vi "Parse U64 Ind Regs.vi"(9 "ECUEvents In":T2, 10 "APU Registers In":T4, 11 "U64":T3[](array[typedef])) -> (1 "ECUEvents Out":T2, 2 "APU Registers Out":T4)   [LabVIEW 2011, in "Engine Sim System Explorer.lvlib"]
uses:
  Engine Sim System Explorer.lvlib
  TypeDefs/APUComp.ctl
  TypeDefs/ECUEventRegs.ctl
  <userlib>/_FPGA Interface Advanced Tools/FPGA Bitfile Utility/TypeDefs/Scalar Register.ctl
  <userlib>/_FPGA Interface Advanced Tools/FPGA Bitfile Utility/FPGA Bitfile Utility.lvlib
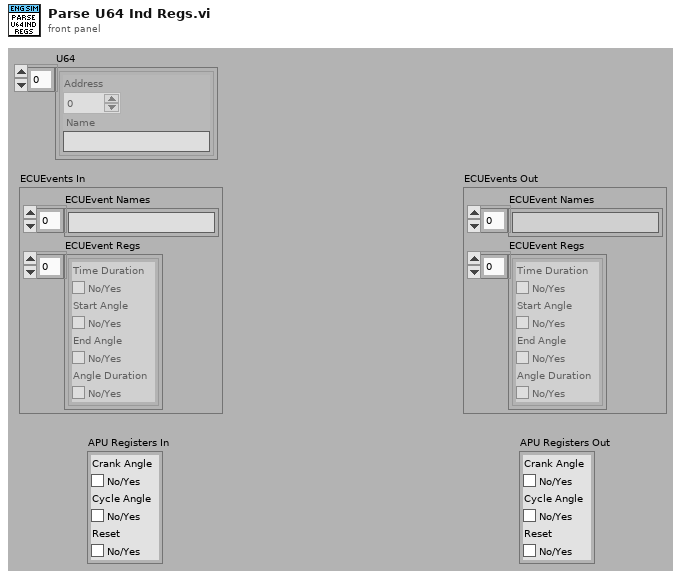
[diagram p1: front panel]
types:
  T1 = typedef "Engine Sim System Explorer.lvlib/ECUEventRegs.ctl" = cluster{"Time Duration":bool, "Start Angle":bool, "End Angle":bool, "Angle Duration":bool}
  T2 = cluster{"ECUEvent Names":string[], "ECUEvent Regs":T1[]}
  T3 = typedef "FPGA Bitfile Utility.lvlib/Scalar Register.ctl" = cluster{"Address":u32, "Name":string}
  T4 = typedef "Engine Sim System Explorer.lvlib/APUComp.ctl" = cluster{"Crank Angle":bool, "Cycle Angle":bool, "Reset":bool}
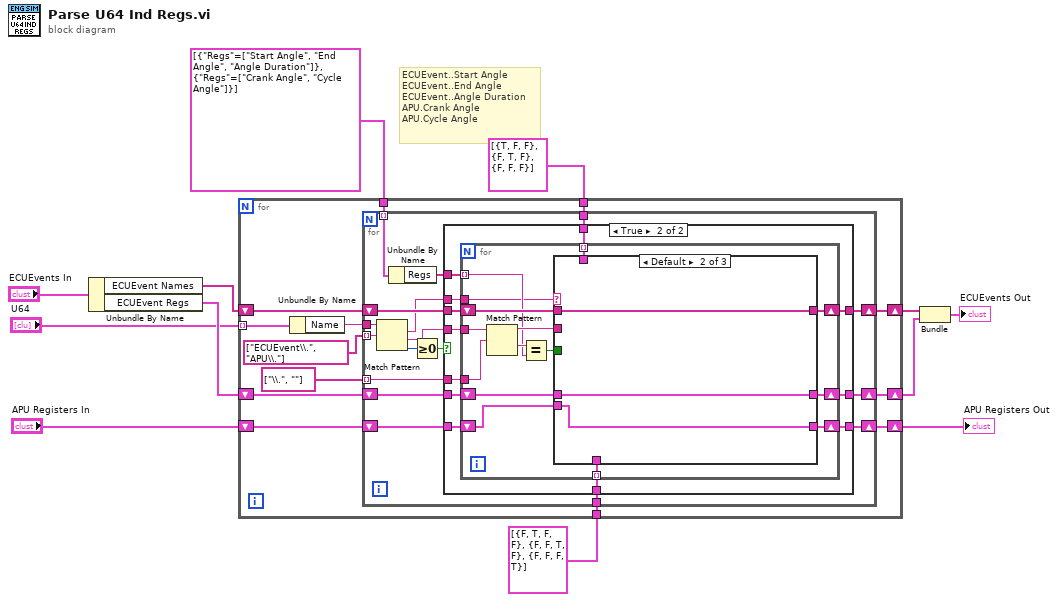
[diagram p0: block diagram]
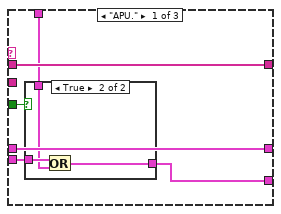
[diagram p3: hidden frame]
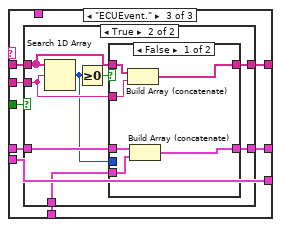
[diagram p5: hidden frame]
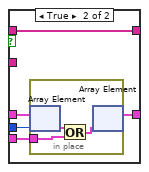
[diagram p7: hidden frame]
diagram:
  # "ECUEvent..Start Angle\nECUEvent..End Angle\nECUEvent..Angle Duration\nAPU.Crank Angle\nAPU.Cycle Angle"
  n1 = Unbundle By Name("ECUEvents In") -> ("ECUEvent Names"=w11:string[], "ECUEvent Regs"=w12:T1[])
  n2 = for {
    tunnel: "U64" -> [w25] mode=indexing
    tunnel: T1[] [{"Time Duration"=FALSE, "Start Angle"=TRUE, "End Angle"=FALSE, "Angle Duration"=FALSE}, {"Time Duration"=FALSE, "Start Angle"=FALSE, "End Angle"=TRUE, "Angle Duration"=FALSE}, {"Time Duration"=FALSE, "Start Angle"=FALSE, "End Angle"=FALSE, "Angle Duration"=TRUE}] -> [w23]
    shift-right: [w22] -> w3
    shift-left: w12 -> [w21]
    shift-right: [w20] -> w4
    shift-left: w11 -> [w19]
    tunnel: cluster{"Regs":string[]}[] [{"Regs"=["Start Angle", "End Angle", "Angle Duration"]}, {"Regs"=["Crank Angle", "Cycle Angle"]}] -> [w17]
    shift-right: [w16] -> w10
    shift-left: "APU Registers In" -> [w15]
    tunnel: T4[] [{"Crank Angle"=TRUE, "Cycle Angle"=FALSE, "Reset"=FALSE}, {"Crank Angle"=FALSE, "Cycle Angle"=TRUE, "Reset"=FALSE}, {"Crank Angle"=FALSE, "Cycle Angle"=FALSE, "Reset"=FALSE}] -> [w14]
    n3 = Unbundle By Name(w25) -> ("Name"=w24:string)
    n4 = for {
      tunnel: w24 -> [w42]
      tunnel: w23 -> [w38]
      tunnel: string[] ["ECUEvent\\.", "APU\\."] -> [w33] mode=indexing
      shift-right: [w35] -> w20
      shift-left: w19 -> [w34]
      shift-right: [w37] -> w22
      shift-left: w21 -> [w36]
      tunnel: w17 -> [w32] mode=indexing
      shift-right: [w29] -> w16
      shift-left: w15 -> [w28]
      tunnel: w14 -> [w27]
      tunnel: string[] ["\\.", ""] -> [w26] mode=indexing
      n5 = Match Pattern(string=w42, regular expression=w33) -> (match substring=w30:string, after substring=w39:string, offset past match=w41:i32)  [unwired: 1 in, 1 out]
      n6 = Unbundle By Name(w32) -> ("Regs"=w31:string[])
      n7 = Greater Or Equal To 0?(x=w41) -> (x >= 0?=w40:bool)
      n8 = case shown="True" w40 {
        tunnel: w39 -> [_ w57]
        tunnel: w38 -> [_ w56]
        tunnel: [w44 w55] -> w37
        tunnel: w36 -> [w44 w54]
        tunnel: [w45 w53] -> w35
        tunnel: w34 -> [w45 w52]
        tunnel: w31 -> [_ w51]
        tunnel: w30 -> [_ w50]
        tunnel: [w43 w49] -> w29
        tunnel: w28 -> [w43 w48]
        tunnel: w27 -> [_ w47]
        tunnel: w26 -> [_ w46]
        frame False {
        }
        frame True {
          n9 = for {
            tunnel: w57 -> [w72]
            tunnel: w56 -> [w68] mode=indexing
            shift-right: [w65] -> w53
            shift-left: w52 -> [w64]
            shift-right: [w67] -> w55
            shift-left: w54 -> [w66]
            tunnel: w51 -> [w63] mode=indexing
            tunnel: w50 -> [w62]
            shift-right: [w61] -> w49
            shift-left: w48 -> [w60]
            tunnel: w47 -> [w59] mode=indexing
            tunnel: w46 -> [w58]
            n10 = Match Pattern(string=w72, regular expression=w58) -> (before substring=w69:string, after substring=w71:string)  [unwired: 1 in, 2 out]
            n11 = Equal?(x=w71, y=w63) -> (x = y?=w70:bool)
            n12 = case shown="Default" w62 {
              tunnel: w70 -> [w73 _ w93]
              tunnel: w69 -> [_ _ w92]
              tunnel: w68 -> [_ _ w91]
              tunnel: [w77 w84 w90] -> w67
              tunnel: w66 -> [w77 w84 w89]
              tunnel: [w78 w85 w88] -> w65
              tunnel: w64 -> [w78 w85 w87]
              tunnel: [w76 w83 w86] -> w61
              tunnel: w60 -> [w75 w83 w86]
              tunnel: w59 -> [w74 _ _]
              frame "APU." {
                n13 = case shown="True" w73 {
                  tunnel: [w79 w82] -> w76
                  tunnel: w75 -> [w79 w81]
                  tunnel: w74 -> [_ w80]
                  frame False {
                  }
                  frame True {
                    n14 = Or(x=w81, y=w80) -> (x .or. y?=w82:T4)
                  }
                }
              }
              frame Default {
              }
              frame "ECUEvent." {
                n15 = case shown="True" w93 {
                  tunnel: w92 -> [_ w98]
                  tunnel: w91 -> [_ w101]
                  tunnel: [w94 w100] -> w90
                  tunnel: w89 -> [w94 w102]
                  tunnel: [w95 w97] -> w88
                  tunnel: w87 -> [w95 w99]
                  frame False {
                  }
                  frame True {
                    n16 = Search 1D Array(1D array=w99, element=w98) -> (index of element=w96:i32)  [unwired: 1 in]
                    n17 = Greater Or Equal To 0?(x=w96) -> (x >= 0?=w103:bool)
                    n18 = case shown="False" w103 {
                      tunnel: w102 -> [w109 w113]
                      tunnel: w101 -> [w108 w111]
                      tunnel: [w107 w110] -> w100
                      tunnel: w99 -> [w106 w114]
                      tunnel: w98 -> [w105 _]
                      tunnel: [w104 w114] -> w97
                      tunnel: w96 -> [_ w112]
                      frame False {
                        n19 = Build Array (concatenate)(w106, w105) -> (w104:string[])
                        n20 = Build Array (concatenate)(w109, w108) -> (w107:T1[])
                      }
                      frame True {
                        n21 = in-place {
                          in-place-border: w111 -> [w116]
                          n22 = in-place-array #1(w113, w112) -> (w117:T1)
                          n23 = Or(x=w117, y=w116) -> (x .or. y?=w115:T1)
                          n24 = in-place-array #1(w115) -> (w110:T1[])  [unwired: 1 out]
                        }
                      }
                    }
                  }
                }
              }
            }
          }
        }
      }
    }
  }
  "APU Registers Out" <- w10
  n25 = Bundle("ECUEvent Names"=w4, "ECUEvent Regs"=w3) -> (→"ECUEvents Out":T2)  [unwired: 1 in]
